vi "Port Session to EU Clusters.vi"(8 "error in":errorcluster, 11 "port sessions":T9 {"session_rx_monitor"."Strobe" items=["FDX_MON_STROBE_DIS", "FDX_MON_STROBE_STOP", "FDX_MON_STROBE_START"]; "session_rx_monitor"."CaptureMode" items=["FDX_MON_SINGLE ", "FDX_MON_CONTINUOUS", "FDX_MON_SELECTIVE", "FDX_MON_RECORDING", "FDX_MON_REROS", "FDX_MON_HMU"]; "session_rx_monitor"."DefaultCronoMode" items=["FDX_RX_DEFAULT_ENA_CNT", "FDX_RX_DEFAULT_MON_ENA_ALL", "FDX_RX_DEFAULT_MON_ENA_GOOD"]}) -> (0 "error out":errorcluster, 2 "Monitor hardware channels":T1={"channel #"=0, "channel handle"=0, "InstrumentHandle_board"=0, "InstrumentHandle_port"=0, "Queue ID"=0, "channel settings"={"Monitor Settings"={"DefaultCronoMode"=0, "GlbMonBufferSizeIn"=0, "CaptureMode"=0, "MaxFileSize MB (1)"=1, "Strobe"=0, "TriggerPosition"=0}, "Rx Board"=0, "Rx Port"=0}, "File Reference"=refnum, "Monitor Log Directory"=""} {"channel settings"."Monitor Settings"."Strobe" items=["FDX_MON_STROBE_DIS", "FDX_MON_STROBE_STOP", "FDX_MON_STROBE_START"]; "channel settings"."Monitor Settings"."CaptureMode" items=["FDX_MON_SINGLE ", "FDX_MON_CONTINUOUS", "FDX_MON_SELECTIVE", "FDX_MON_RECORDING", "FDX_MON_REROS", "FDX_MON_HMU"]; "channel settings"."Monitor Settings"."DefaultCronoMode" items=["FDX_RX_DEFAULT_ENA_CNT", "FDX_RX_DEFAULT_MON_ENA_ALL", "FDX_RX_DEFAULT_MON_ENA_GOOD"]}, 3 "Tx hardware channels":T4 {"channel settings"."Frame Array"."Raw Frame" format="%.0x"; "channel settings"."Frame Array"."Frame Configuration"."interfaceID" format="%.0b"; "channel settings"."Frame Array"."HeaderInfo"."NetSelect" items=["FDX_TX_FRAME_DLY_A"=0, "FDX_TX_FRAME_DLY_B"=1, "FDX_TX_FRAME_BOTH "=3, "FDX_TX_FRAME_ONLY_A"=4, "FDX_TX_FRAME_ONLY_B "=5]; "channel settings"."Frame Array"."HeaderInfo"."FrameStartMode" items=["FDX_TX_FRAME_START_IFG", "FDX_TX_FRAME_START_PGWT", "FDX_TX_FRAME_START_TRG"]; "channel settings"."Frame Array"."HeaderInfo"."PhysErrorInjection" items=["FDX_TX_FRAME_ERR_OFF"=0, "FDX_TX_FRAME_ERR_CRC"=1, "FDX_TX_FRAME_ERR_ALI"=2, "FDX_TX_FRAME_ERR_PRE"=4, "FDX_TX_FRAME_ERR_PHY"=8]; "channel settings"."Frame Array"."HeaderInfo"."SequenceNumberInit" items=["FDX_TX_FRAME_SEQ_INIT_AUTO"=65535]; "channel settings"."Frame Array"."HeaderInfo"."SequenceNumberOffset" items=["FDX_TX_FRAME_SEQ_OFFS_AUTO "=65535]; "channel settings"."Frame Array"."HeaderInfo"."PayloadGenerationMode" items=["FDX_TX_FRAME_PGM_USER"=0, "FDX_TX_FRAME_PGM_IP_PART"=1, "FDX_TX_FRAME_PGM_IP_FULL"=2, "FDX_TX_FRAME_PGM_IP_PART_TT"=10, "FDX_TX_FRAME_PGM_IP_FULL_TT"=20]; "channel settings"."Frame Array"."HeaderInfo"."PayloadBufferMode" items=["FDX_TX_FRAME_PBM_STD", "FDX_TX_FRAME_PBM_MAC", "FDX_TX_FRAME_PBM_UDP"]})   [LabVIEW 2020, in "AIM ARINC 664 Scripting.lvlib"]
uses:
  AIM ARINC 664 Scripting.lvlib
  AIM LabVIEW src/src/_controls/session_monitor_config.ctl
  AIM LabVIEW src/src/AIM664LV.lvlib
  Engine/Implementation/Monitor Execution Unit/channel_settings_rx.ctl
  Engine/Implementation/Monitor Execution Unit/Monitor Execution Unit.lvclass
  Engine/Implementation/Monitor Execution Unit/hardware_channels_rx.ctl
  AIM LabVIEW src/src/_controls/queue_header_generic.ctl
  AIM LabVIEW src/src/_controls/queue_data_full.ctl
  Engine/Implementation/Frame.ctl
  Engine/Implementation/Tx Execution Unit/channel_settings_tx.ctl
  Engine/Implementation/Tx Execution Unit/Tx Generic Execution Unit.lvclass
  Engine/Implementation/Tx Execution Unit/hardware_channels_tx.ctl
  Shared/session_tx_generic.ctl
  Shared/session_rx_monitor.ctl
  Shared/Port Session Configuration.ctl
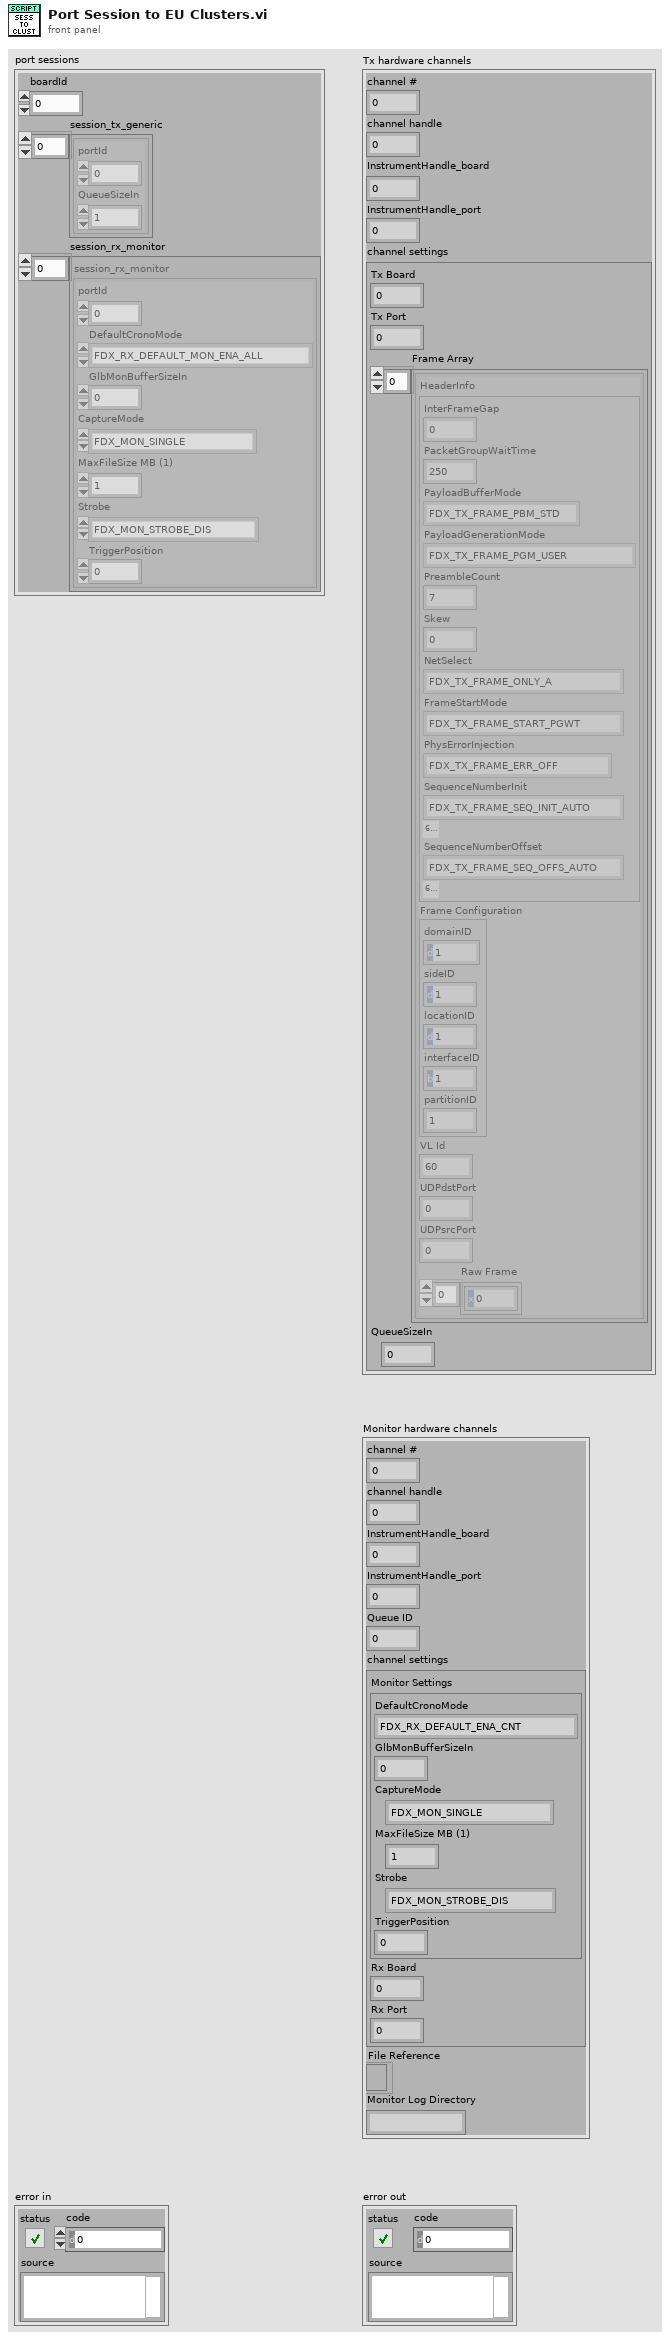
[diagram p1: front panel]
types:
  T1 = typedef "AIM ARINC 664 Engine.lvlib/Implementation.lvlib/Monitor Execution Unit.lvclass/hardware_channels_rx.ctl" = cluster{"channel #":u16, "channel handle":u64, "InstrumentHandle_board":u32, "InstrumentHandle_port":u32, "Queue ID":u32, "channel settings":T2, "File Reference":refnum<file>, "Monitor Log Directory":string}
  T2 = typedef "AIM ARINC 664 Engine.lvlib/Implementation.lvlib/Monitor Execution Unit.lvclass/channel_settings_rx.ctl" = cluster{"Monitor Settings":T3, "Rx Board":u32, "Rx Port":u32}
  T3 = typedef "AIM664LV.lvlib/session_monitor_config.ctl" = cluster{"DefaultCronoMode":u32, "GlbMonBufferSizeIn":u32, "CaptureMode":u32, "MaxFileSize MB (1)":u32, "Strobe":u32, "TriggerPosition":u32}
  T4 = typedef "AIM ARINC 664 Engine.lvlib/Implementation.lvlib/Tx Generic Execution Unit.lvclass/hardware_channels_tx.ctl" = cluster{"channel #":u16, "channel handle":u64, "InstrumentHandle_board":u32, "InstrumentHandle_port":u32, "channel settings":T5}
  T5 = typedef "AIM ARINC 664 Engine.lvlib/Implementation.lvlib/Tx Generic Execution Unit.lvclass/channel_settings_tx.ctl" = cluster{"Tx Board":u32, "Tx Port":u32, "Frame Array":T6[], "QueueSizeIn":u32}
  T6 = typedef "Frame.ctl" = cluster{"HeaderInfo":T7, "Frame Configuration":T8, "VL Id":u16, "UDPdstPort":u16, "UDPsrcPort":u16, "Raw Frame":u8[]}
  T7 = typedef "AIM664LV.lvlib/queue_header_generic.ctl" = cluster{"InterFrameGap":u32, "PacketGroupWaitTime":u32, "PayloadBufferMode":u8, "PayloadGenerationMode":u8, "PreambleCount":u8, "Skew":u32, "NetSelect":u8, "FrameStartMode":u8, "PhysErrorInjection":u32, "SequenceNumberInit":u16, "SequenceNumberOffset":u16}
  T8 = typedef "AIM664LV.lvlib/queue_data_full.ctl" = cluster{"domainID":u8, "sideID":u8, "locationID":u8, "interfaceID":u8, "partitionID":u8}
  T9 = typedef "Port Session Configuration.ctl" = cluster{"boardId":u32, "session_tx_generic":T10[], "session_rx_monitor":T11[]}
  T10 = typedef "session_tx_generic.ctl" = cluster{"portId":u32, "QueueSizeIn":u32}
  T11 = typedef "session_rx_monitor.ctl" = cluster{"portId":u32, "DefaultCronoMode":u32, "GlbMonBufferSizeIn":u32, "CaptureMode":u32, "MaxFileSize MB (1)":u32, "Strobe":u32, "TriggerPosition":u32}
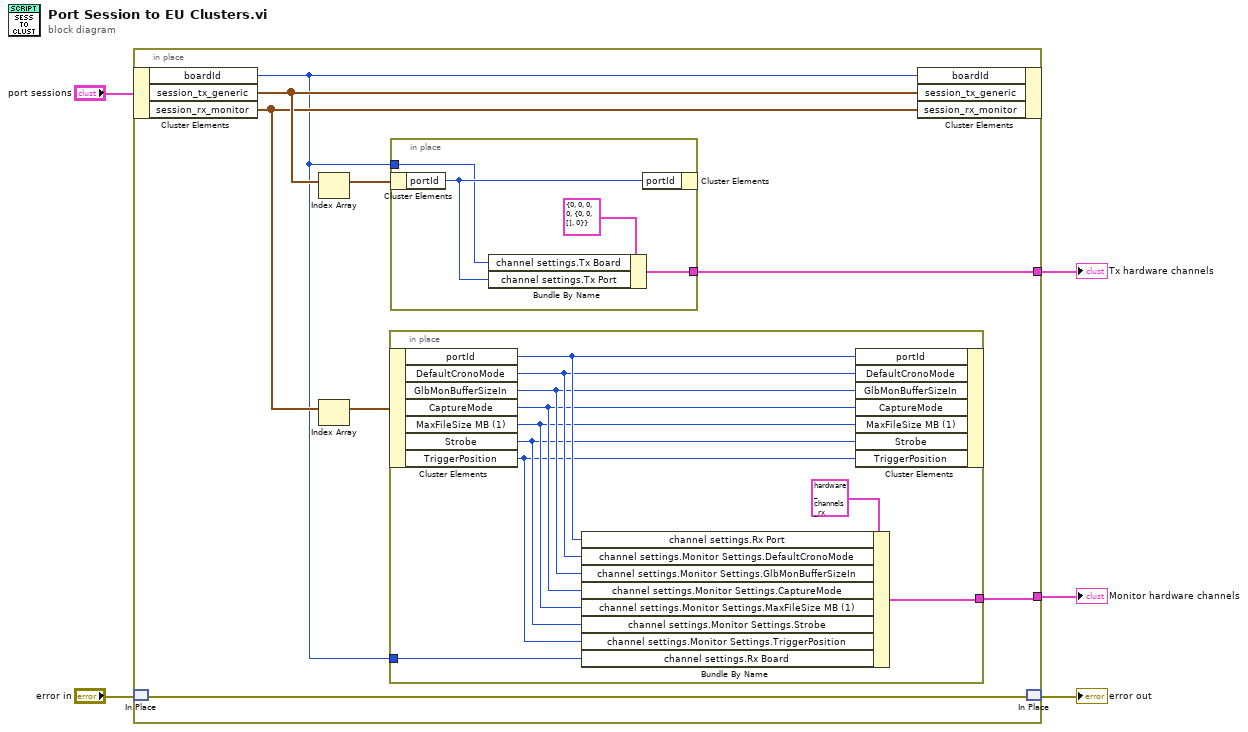
[diagram p0: block diagram]
diagram:
  n1 = in-place {
    in-place-border: [w9] -> w4
    in-place-border: [w8] -> w3
    n2 = in-place-cluster #1("port sessions") -> ("boardId"=w6:u32, "session_tx_generic"=w13:T10[], "session_rx_monitor"=w12:T11[])
    n3 = in-place-match #2("error in") -> (w7:errorcluster)
    n4 = Index Array(array=w13) -> (element=w11:T10)  [unwired: 1 in]
    n5 = Index Array(array=w12) -> (element=w10:T11)  [unwired: 1 in]
    n6 = in-place {
      in-place-border: [w19] -> w8
      in-place-border: w6 -> [w18]
      n7 = in-place-cluster #3(w10) -> ("portId"=w26:u32, "DefaultCronoMode"=w25:u32, "GlbMonBufferSizeIn"=w24:u32, "CaptureMode"=w23:u32, "MaxFileSize MB (1)"=w22:u32, "Strobe"=w21:u32, "TriggerPosition"=w20:u32)
      n8 = Bundle By Name(cluster=T1 {"channel #"=0, "channel handle"=0, "InstrumentHandle_board"=0, "InstrumentHandle_port"=0, "Queue ID"=0, "channel settings"={"Monitor Settings"={"DefaultCronoMode"=0, "GlbMonBufferSizeIn"=0, "CaptureMode"=0, "MaxFileSize MB (1)"=1, "Strobe"=0, "TriggerPosition"=0}, "Rx Board"=0, "Rx Port"=0}, "File Reference"=refnum, "Monitor Log Directory"=""} ("hardware channels"), "channel settings.Rx Port"=w26, "channel settings.Monitor Settings.DefaultCronoMode"=w25, "channel settings.Monitor Settings.GlbMonBufferSizeIn"=w24, "channel settings.Monitor Settings.CaptureMode"=w23, "channel settings.Monitor Settings.MaxFileSize MB (1)"=w22, "channel settings.Monitor Settings.Strobe"=w21, "channel settings.Monitor Settings.TriggerPosition"=w20, "channel settings.Rx Board"=w18) -> (w19:T1)
      n9 = in-place-cluster #3("portId"=w26, "DefaultCronoMode"=w25, "GlbMonBufferSizeIn"=w24, "CaptureMode"=w23, "MaxFileSize MB (1)"=w22, "Strobe"=w21, "TriggerPosition"=w20) -> ()  [unwired: 1 out]
    }
    n10 = in-place {
      in-place-border: w6 -> [w15]
      in-place-border: [w14] -> w9
      n11 = in-place-cluster #4(w11) -> ("portId"=w16:u32)
      n12 = Bundle By Name(cluster=T4 {"channel #"=0, "channel handle"=0, "InstrumentHandle_board"=0, "InstrumentHandle_port"=0, "channel settings"={"Tx Board"=0, "Tx Port"=0, "Frame Array"=[], "QueueSizeIn"=0}} ("hardware channels"), "channel settings.Tx Board"=w15, "channel settings.Tx Port"=w16) -> (w14:T4)
      n13 = in-place-cluster #4("portId"=w16) -> ()  [unwired: 1 out]
    }
    n14 = in-place-cluster #1("boardId"=w6, "session_tx_generic"=w13, "session_rx_monitor"=w12) -> ()  [unwired: 1 out]
    n15 = in-place-match #2(w7) -> (→"error out":errorcluster)
  }
  "Tx hardware channels" <- w4
  "Monitor hardware channels" <- w3
